vi "WaitEventDataExamplevi.vi"() -> ()   [LabVIEW 2010]
uses:
  <vilib>/MDSplus/Library/MDSplus.lvlib
panel:
  out "Event Data":sgl format="%.3f"
  in  "Event Name":string
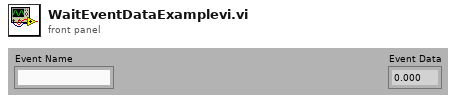
[diagram p1: front panel]
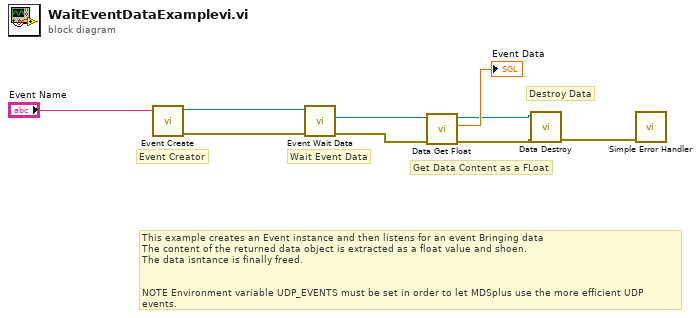
[diagram p0: block diagram]
diagram:
  # "This example creates an Event instance and then listens for an event Bringing data\nThe content of the returned data object is extracted as a float value and shoen. \nThe data isntance is finally freed.\n\n\nNOTE Environment variable UDP_EVENTS must be set in order to let MDSplus use the more efficient UDP events."
  # "Destroy Data"
  # "Get Data Content as a FLoat"
  # "Wait Event Data"
  # "Event Creator"
  n1 = call <vilib>:"Event Create.vi"("Event name"="Event Name") -> ("error out"=w7:errorcluster, "Event DVR out"=w8:refnum<data-value>)  [unwired: 9 in]
  n2 = call <vilib>:"Event Wait Data.vi"("error in (no error)"=w7, "Event DVR in"=w8) -> ("error out"=w5:errorcluster, "Data out"=w6:refnum<data-value>)  [unwired: 7 in, 1 out]
  n3 = call <vilib>:"Data Get Float.vi"("error in (no error)"=w5, "Data DVR in"=w6) -> ("error out"=w2:errorcluster, "SGL out"=→"Event Data":sgl, "Data DVR out"=w3:refnum<data-value>)  [unwired: 7 in]
  n4 = call <vilib>:"Data Destroy.vi"("error in (no error)"=w2, "Data DVR in"=w3) -> ("error out"=w1:errorcluster)  [unwired: 9 in]
  n5 = call <vilib>:"Simple Error Handler.vi"("error in (no error)"=w1) -> ()  [unwired: 4 in, 5 out]
